vi "Power Spectrum Density Global.vi"() -> ()   [LabVIEW 2023, in "Power Spectrum Density.lvlib" / "Power Spectrum Density.lvclass"]
uses:
  Power Spectrum Density.lvclass
  <vilib>/measure/maspectr.llb/Power Spectrum and PSD Export Mode.ctl
  <vilib>/Analysis/4window.llb/windowTd.ctl
  <vilib>/Analysis/NI_AALPro.lvlib
  <vilib>/measure/NI_MAPro.lvlib
panel:
  in  "Number of Samples":string="Number of Samples"
  in  "Weighting mode strings":string[](array[string])=["Linear", "Exponential"]
  in  "Averaging mode strings":string[](array[string])=["No averaging", "Vector averaging", "RMS averaging", "Peak hold"]
  in  "Window values":T1[](array[typedef])=[0, 1, 2, 3, 4, 5, 6, 7, 8, 9, 11, 30, 31, 32, 33, 34, 60, 61, 62] items=["Rectangle"=0, "Hanning"=1, "Hamming"=2, "Blackman-Harris"=3, "Exact Blackman"=4, "Blackman"=5, "Flat Top"=6, "4 Term B-Harris "=7, "7 Term B-Harris"=8, "Low Sidelobe"=9, "Blackman Nuttall"=11, "Triangle"=30, "Bartlett-Hanning"=31, "Bohman"=32, "Parzen"=33, "Welch"=34, "Kaiser"=60, "Dolph-Chebyshev"=61, "Gaussian"=62]
  in  "Export mode values":T2[](array[typedef])=[0, 1] items=["Power Spectrum", "Power Spectral Density"]
  in  "Weighting mode values":enum16{"Linear", "Exponential"}[](array[ring])=[enum."Linear", enum."Exponential"]
  in  "Averaging mode values":T3(array[ring])=[enum."No averaging", enum."Vector averaging", enum."RMS averaging", enum."Peak hold"]
  in  "Window parameter":string="Window parameter"
  in  "Number of averages":string="Number of averages"
  in  "Weighting mode":string="Weighting mode"
  in  "Window Strings":string[](array[string])=["Rectangle", "Hanning", "Hamming", "Blackman-Harris", "Exact Blackman", "Blackman", "Flat Top", "4 Term B-Harris", "7 Term B-Harris", "Low Sidelobe", "Blackman Nuttal", "Triangle", "Barlett-Hanning", "Bohman", "Parzen", "Welch", "Kaiser", "Dolph-Chebyshev", "Gaussian"]
  in  "Averaging mode":string="Averaging mode"
  in  "dB":string="dB"
  in  "Window":string="Window"
  in  "Export mode strings":string[](array[string])=["Power Spectrum", "Power Spectral Density"]
  in  "Export mode":string="Export mode"
  in  "Show PSD Window":string="Show Power Spectrum Density Window"
  in  "Select Channel":string="Select Channel"
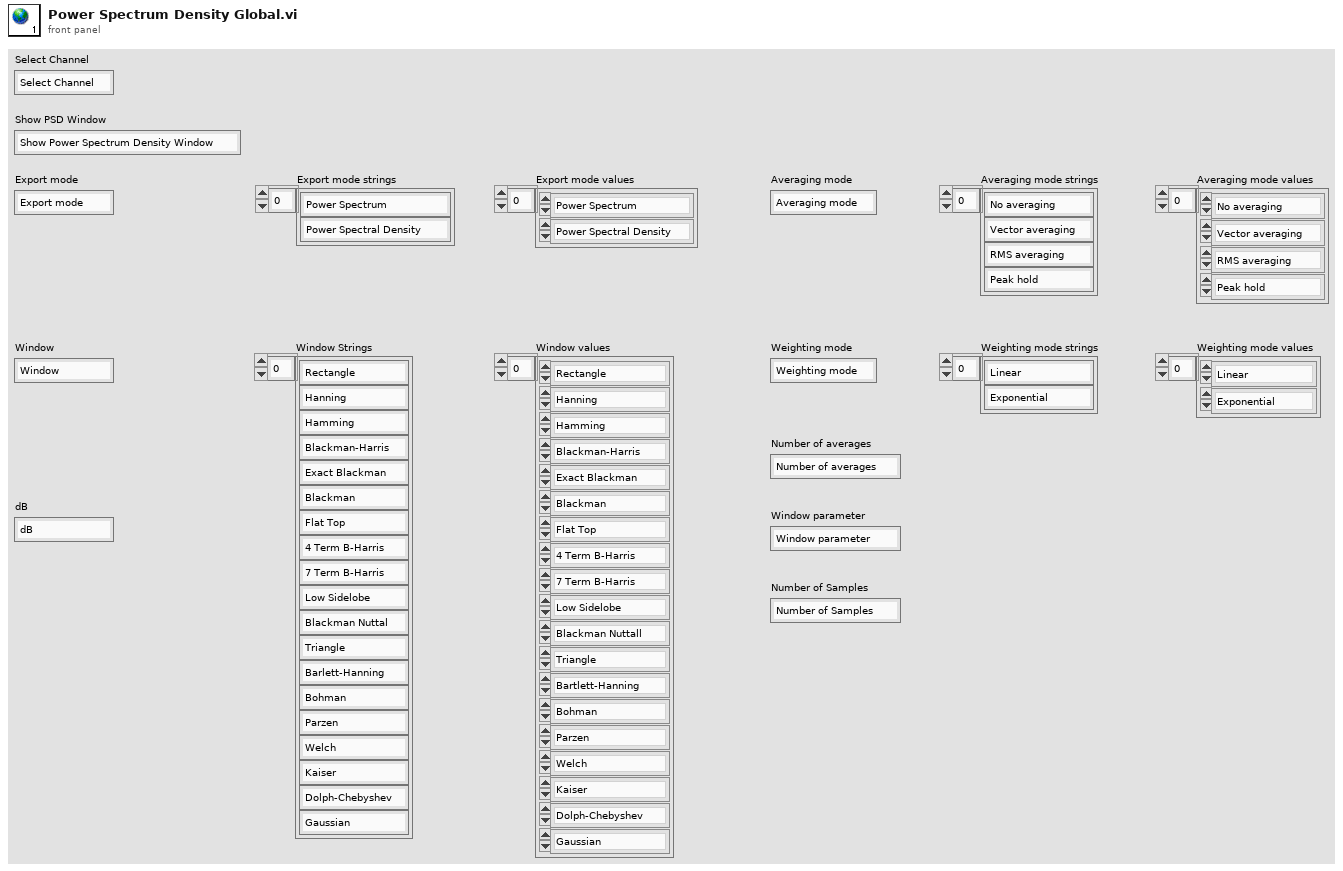
[diagram p1: front panel]
types:
  T1 = typedef "NI_AALPro.lvlib/windowTd.ctl" = u32
  T2 = typedef "NI_MAPro.lvlib/Power Spectrum and PSD Export Mode.ctl" = u16
  T3 = enum16{"No averaging", "Vector averaging", "RMS averaging", "Peak hold"}[]
diagram:
